vi "每周自动更新循环.vi"   [LabVIEW 2016, in "数据传输系统-05.lvlib"]
uses:
  <vilib>/ptbypt/NI_PtbyPt.lvlib
types:
  T1 = enum16{"关闭", "星期日", "星期一", "星期二", "星期三", "星期四", "星期五", "星期六"}
  T2 = typedef "LVDateTimeRec.ctl" = cluster{"秒数的小数部分":dbl, "秒":i32, "分":i32, "时":i32, "日":i32, "月":i32, "年":i32, "天数（周）":i32, "天数（年）":i32, "DST":i32}
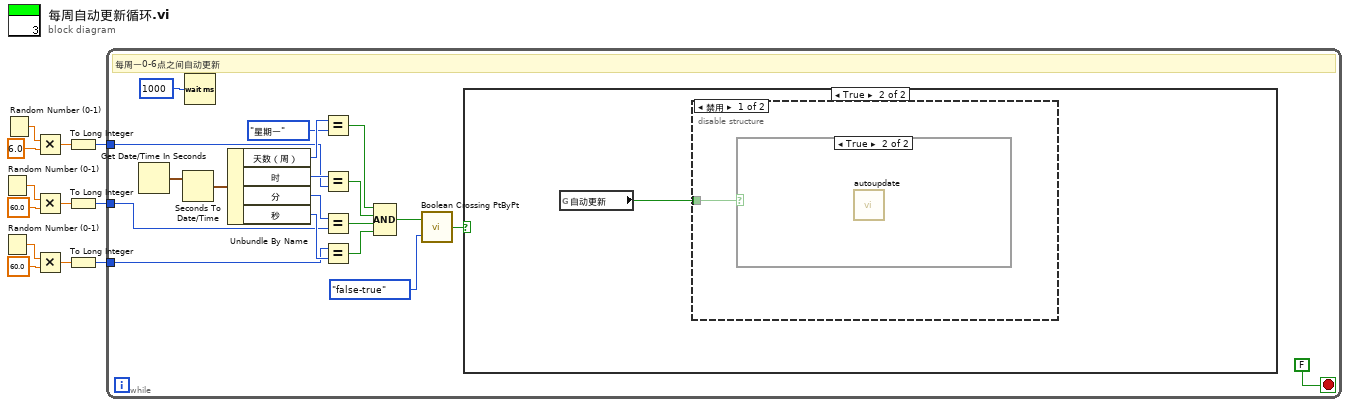
[diagram p0: block diagram]
diagram:
  n1 = Random Number (0-1)() -> (number: 0 to 1=w4:dbl)
  n2 = Random Number (0-1)() -> (number: 0 to 1=w5:dbl)
  n3 = Random Number (0-1)() -> (number: 0 to 1=w1:dbl)
  n4 = Multiply(x=w1, y=6.0) -> (x*y=w7:dbl)
  n5 = Multiply(x=w4, y=60.0) -> (x*y=w9:dbl)
  n6 = Multiply(x=w5, y=60.0) -> (x*y=w11:dbl)
  n7 = To Long Integer(number=w7) -> (32bit integer=w8:i32)
  n8 = To Long Integer(number=w9) -> (32bit integer=w10:i32)
  n9 = To Long Integer(number=w11) -> (32bit integer=w12:i32)
  n10 = while {
    tunnel: w8 -> [w20]
    tunnel: w10 -> [w15]
    tunnel: w12 -> [w14]
    stop <- FALSE stop-if-true
    # "每周一0-6点之间自动更新"
    n11 = Get Date/Time In Seconds() -> (seconds since 1Jan1904=w29:timestamp)
    n12 = Seconds To Date/Time(time stamp (now)=w29) -> (date time rec=w25:T2)  [unwired: 1 in]
    n13 = Wait (ms)(milliseconds to wait=u32 1000 ("等待时间（毫秒）")) -> ()  [unwired: 1 out]
    n14 = Unbundle By Name(w25) -> ("天数（周）"=w28:i32, "时"=w22:i32, "分"=w19:i32, "秒"=w17:i32)
    n15 = Equal?(x=w28, y=T1."星期一" ("重发日期")) -> (x = y?=w27:bool)
    n16 = Equal?(x=w22, y=w20) -> (x = y?=w26:bool)
    n17 = Equal?(x=w19, y=w15) -> (x = y?=w18:bool)
    n18 = Equal?(x=w14, y=w17) -> (x = y?=w16:bool)
    n19 = Compound Arithmetic op=AND ("复合运算")(w27, w26, w18, w16) -> (w24:bool)
    n20 = call <vilib>:"Boolean Crossing PtByPt.vi"("direction"=enum16{"either", "false-true", "true-false"}."false-true", "input"=w24) -> ("crossing"=w13:bool)  [unwired: 1 in]
    n21 = case shown="True" w13 {
      frame False {
      }
      frame True {
        n22 = global read "断电保存全局.vi" "自动更新"() -> (w32:bool)
        n23 = disable-structure shown="禁用" {
          disable-tunnel: w32 -> [w33 _]
          frame Disabled {
            n24 = case shown="True" w33 {
              frame False {
              }
              frame True {
                n25 = call "autoupdate.vi"() -> ()  [unwired: 12 in]
              }
            }
          }
          frame Enabled {
          }
        }
      }
    }
  }
